vi "test Append Block.vi"(8 "error in (no error)":errorcluster, 11 "TestCase in":refnum<class "Test_Blob.lvclass">) -> (0 "error out":errorcluster, 3 "TestCase out":refnum<class "Test_Blob.lvclass">)   [LabVIEW 2015, in "Test_Blob.lvclass"]
uses:
  Test_Blob.lvclass
  Blob Storage/Blob Type.ctl
  Global Parameters.vi
  Core/Session/Session.lvclass
  Blob Storage/NI_Azure_Blob.lvlib
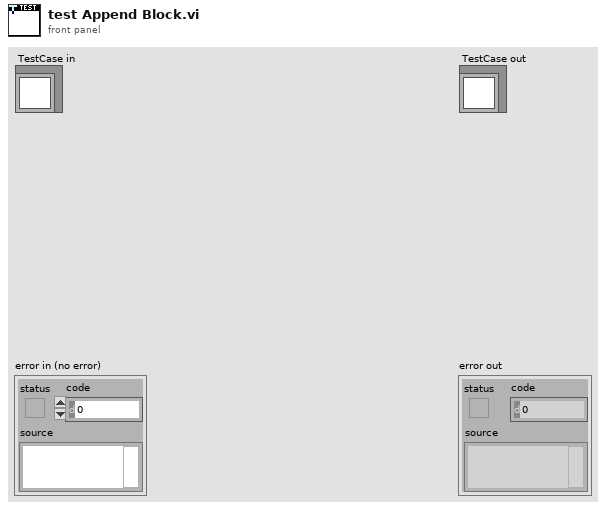
[diagram p1: front panel]
types:
  T1 = typedef "NI_Azure_Blob.lvlib/Blob Type.ctl" = enum16{"BlockBlob", "PageBlob", "AppendBlob"}
  T2 = typedef "NI_Azure_Core.lvlib/Session.lvclass/Azure Credentials.ctl" = cluster{"Storage Account Name":string, "Access Key":string}
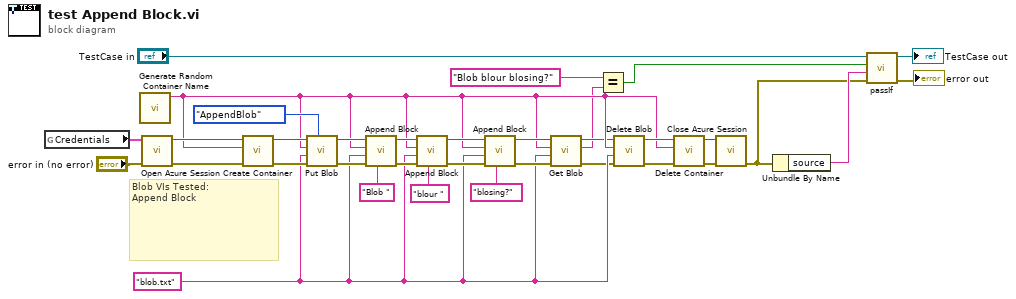
[diagram p0: block diagram]
diagram:
  w9 = "blob.txt"
  # "Blob VIs Tested:\nAppend Block"
  n1 = global read "Global Parameters.vi" "Credentials"() -> (w24:T2)
  n2 = call "Generate Random Container Name.vi"() -> ("Random Container Name"=w10:string)  [unwired: 11 in]
  n3 = call "Open Azure Session.vi"("error in (no error)"="error in (no error)", "Credentials"=w24) -> ("error out"=w25:errorcluster, "Azure Session"=w22:refnum<class "Session.lvclass">)  [unwired: 8 in]
  n4 = call "Create Container.vi"("error in (no error)"=w25, "Container"=w10, "Azure Session in"=w22) -> ("error out"=w30:errorcluster, "Azure Session out"=w29:refnum<class "Session.lvclass">)  [unwired: 7 in]
  n5 = call "Put Blob.vi"("Blob type"=Blob_Type."AppendBlob", "error in (no error)"=w30, "Blob"=w9, "Container"=w10, "Azure Session in"=w29) -> ("error out"=w15:errorcluster, "Azure Session out"=w14:refnum<class "Session.lvclass">)  [unwired: 5 in]
  n6 = call "Append Block.vi"("Blob Content"="Blob ", "error in (no error)"=w15, "Blob"=w9, "Container"=w10, "Azure Session in"=w14) -> ("error out"=w18:errorcluster, "Azure Session out"=w16:refnum<class "Session.lvclass">)  [unwired: 5 in]
  n7 = call "Append Block.vi"("Blob Content"="blour ", "error in (no error)"=w18, "Blob"=w9, "Container"=w10, "Azure Session in"=w16) -> ("error out"=w17:errorcluster, "Azure Session out"=w12:refnum<class "Session.lvclass">)  [unwired: 5 in]
  n8 = call "Append Block.vi"("Blob Content"="blosing?", "error in (no error)"=w17, "Blob"=w9, "Container"=w10, "Azure Session in"=w12) -> ("error out"=w13:errorcluster, "Azure Session out"=w11:refnum<class "Session.lvclass">)  [unwired: 5 in]
  n9 = call "Get Blob.vi"("error in (no error)"=w13, "Blob"=w9, "Container"=w10, "Azure Session in"=w11) -> ("error out"=w8:errorcluster, "Blob Content"=w6:string, "Azure Session out"=w7:refnum<class "Session.lvclass">)  [unwired: 5 in]
  n10 = Equal?(x="Blob blour blosing?" ("y"), y=w6) -> (x = y?=w4:bool)
  n11 = call "Delete Blob.vi"("error in (no error)"=w8, "Blob"=w9, "Container"=w10, "Azure Session in"=w7) -> ("error out"=w28:errorcluster, "Azure Session out"=w27:refnum<class "Session.lvclass">)  [unwired: 6 in]
  n12 = call "Delete Container.vi"("error in (no error)"=w28, "Container"=w10, "Azure Session in"=w27) -> ("error out"=w23:errorcluster, "Azure Session out"=w19:refnum<class "Session.lvclass">)  [unwired: 7 in]
  n13 = call "Close Azure Session.vi"("error in (no error)"=w23, "Azure Session"=w19) -> ("error out"=w20:errorcluster)  [unwired: 9 in]
  n14 = Unbundle By Name(w20) -> ("source"=w31:string)
  n15 = call-dynamic "passIf.vi"("error in (no error)"=w20, "message (\"\")"=w31, "pass"=w4, "TestCase in"="TestCase in") -> ("error out"=→"error out":errorcluster, "TestCase out"=→"TestCase out":refnum<class "Test_Blob.lvclass">)  [unwired: 6 in]
